vi "Revision Query.vi"(7 "Pump ID (0:A)":T1, 8 "error in (no error)":errorcluster, 11 "VISA resource in":refnum<visa-resource-name>) -> (0 "error out":errorcluster, 1 "Firmware Revision":i32, 2 "Instrument Driver Revision":string, 3 "VISA resource out":refnum<visa-resource-name>)   [LabVIEW 2020, in "Global FIA milliGAT.lvlib"]
doc: "Queries the current instrument firmware revision and instrument driver revision.\n\nRefer to the Readme file for detailed driver information including modification history."
uses:
  <instrlib>/RxnRover/Global FIA milliGAT 3.14/Global FIA milliGAT.lvlib
  <instrlib>/RxnRover/Global FIA milliGAT 3.14/Public/Utility/Pump Address.ctl
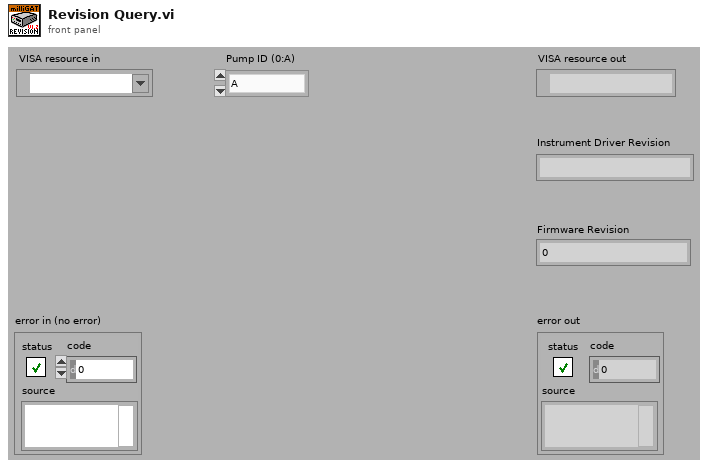
[diagram p1: front panel]
types:
  T1 = typedef "Global FIA milliGAT.lvlib/Pump Address.ctl" = enum16{"A", "B", "C", "D", "E", "F", "G", "H", "I", "J", "K", "L", "M", "N", "O", "P", "Q", "R", "S", "T", "U", "V", "W", "X", "Y", "Z", "a", "b", "c", "d", "e", "f", "g", "h", "i", "j", "k", "l", "m", "n", "o", "p", "q", "r", "s", "t", "u", "v", "w", "x", "y", "z", "0", "1", "2", "3", "4", "5", "6", "7", "8", "9"}
  T2 = enum32{"invalid app kind", "Development System", "Run Time System", "Student Edition", "Embedded LabVIEW", "Evaluation", "Custom"}
  T3 = cluster{"Major":u16, "Minor":u16, "Fix":u16, "Build":u16}
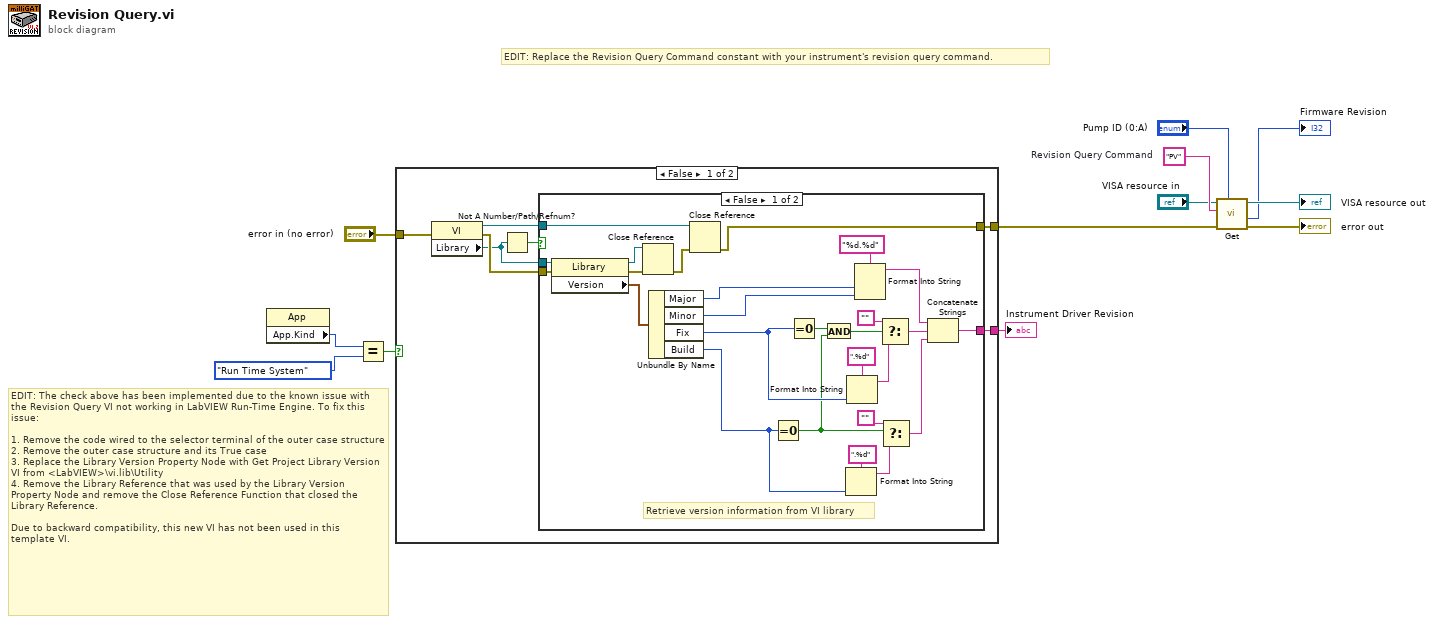
[diagram p0: block diagram]
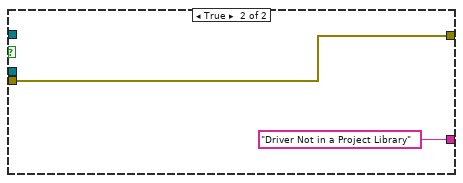
[diagram p2: hidden frame]
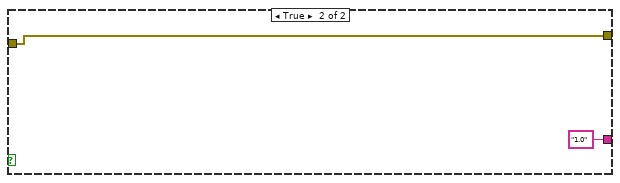
[diagram p3: hidden frame]
diagram:
  w7 = "PV"  # Revision Query Command
  # "EDIT: The check above has been implemented due to the known issue with the Revision Query VI not working in LabVIEW Run-Time Engine. To fix this issue:\n\n1. Remove the code wired to the selector terminal of the outer case structure\n2. Remove the outer case structure and its True case\n3. Replace the Library Version Property Node with Get Project Library Version VI from <LabVIEW>\\vi.lib\\Utility\n4. Remove the Library Reference that was used by the Library Version Property Node and remove the Close Reference Function that closed the Library Reference.\n\nDue to backward compatibility, this new VI has not been used in this template VI."
  # "EDIT: Replace the Revision Query Command constant with your instrument's revision query command."
  n1 = property class="App"() -> ("App.Kind"=w9:T2)  [unwired: 2 in, 2 out]
  n2 = Equal?(x=w9, y=T2."Run Time System" ("Application:Kind")) -> (x = y?=w10:bool)
  n3 = case shown="False" w10 {
    tunnel: [w15 "1.0"] -> w12
    tunnel: "error in (no error)" -> [w14 w48]
    tunnel: [w13 w48] -> w5
    frame False {
      n4 = property class="VI"(error in=w14) -> (reference out=w19:refnum<vi>, error out=w18:errorcluster, "Library"=w17:refnum<vi>)  [unwired: 1 in]
      n5 = Not A Number/Path/Refnum?(number/path/refnum=w17) -> (NaN/Path/Refnum?=w16:bool)
      n6 = case shown="False" w16 {
        tunnel: w19 -> [w42 _]
        tunnel: w18 -> [w27 w47]
        tunnel: [w22 w47] -> w13
        tunnel: [w21 "Driver Not in a Project Library"] -> w15
        tunnel: w17 -> [w20 _]
        frame False {
          # "Retrieve version information from VI library"
          n7 = property class="Library"(reference=w20, error in=w27) -> (reference out=w44:refnum<vi>, error out=w45:errorcluster, "Version"=w41:T3)
          n8 = Close Reference(reference=w44, error in (no error)=w45) -> (error out=w43:errorcluster)
          n9 = Unbundle By Name(w41) -> ("Major"=w30:u16, "Minor"=w29:u16, "Fix"=w26:u16, "Build"=w28:u16)
          n10 = Close Reference(reference=w42, error in (no error)=w43) -> (error out=w22:errorcluster)
          n11 = Equal To 0?(x=w28) -> (x = 0?=w24:bool)
          n12 = Equal To 0?(x=w26) -> (x = 0?=w25:bool)
          n13 = And(x=w25, y=w24) -> (x .and. y?=w23:bool)
          n14 = Format Into String(format string=".%d", w28) -> (resulting string=w34:string)  [unwired: 2 in, 1 out]
          n15 = Format Into String(format string=".%d", w26) -> (resulting string=w38:string)  [unwired: 2 in, 1 out]
          n16 = Format Into String(format string="%d.%d", w30, w29) -> (resulting string=w36:string)  [unwired: 2 in, 1 out]
          n17 = Select(t="", s=w23, f=w38) -> (s? t:f=w35:string)
          n18 = Select(t="", s=w24, f=w34) -> (s? t:f=w31:string)
          n19 = Concatenate Strings(w36, w35, w31) -> (w21:string)
        }
        frame True {
        }
      }
    }
    frame True {
    }
  }
  "Instrument Driver Revision" <- w12
  n20 = call <instrlib>:"Get.vi"("Pump ID (0:A)"="Pump ID (0:A)", "error in (no error)"=w5, "Parameter"=w7, "VISA resource in"="VISA resource in") -> ("error out"=→"error out":errorcluster, "Value"=→"Firmware Revision":i32, "VISA resource out"=→"VISA resource out":refnum<visa-resource-name>)  [unwired: 5 in]
